vi "Get Authority.vi"(8 "error in (no error)":errorcluster, 11 "URI in":refnum<class "URI.lvclass">) -> (0 "error out":errorcluster, 2 "Authority":string, 3 "URI out":refnum<class "URI.lvclass">)   [LabVIEW 2020, in "IO.lvlib" / "URI.lvclass"]
uses:
  URI.lvclass
  URI.lvclass/URI.ctl
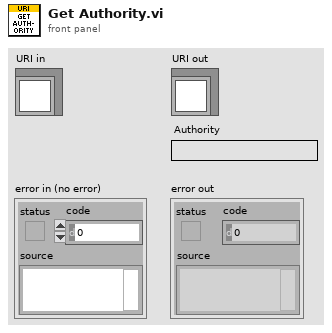
[diagram p1: front panel]
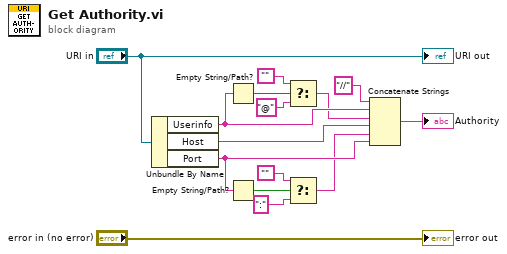
[diagram p0: block diagram]
diagram:
  n1 = Unbundle By Name("URI in") -> ("Userinfo"=w10:string, "Host"=w7:string, "Port"=w3:string)
  n2 = Empty String/Path?(string/path=w10) -> (empty?=w13:bool)
  n3 = Empty String/Path?(string/path=w3) -> (empty?=w4:bool)
  n4 = Select(t="", s=w13, f="@") -> (s? t:f=w8:string)
  n5 = Select(t="", s=w4, f=":") -> (s? t:f=w2:string)
  n6 = Concatenate Strings("//" ("string"), w10, w8, w7, w2, w3) -> (→"Authority":string)
  "error out" <- "error in (no error)"
  "URI out" <- "URI in"
